vi "CRYCalc Wave & Value Unit.vi"(8 "Work in":u16(slide), 9 "Operator":u16(ring) items=["+", "--", "x", "/"], 10 "Value in":T1={"Name"="", "Curve"=[], "X data"=1, "Y data"=1, "Z data"=1, "X axis"=0, "Y axis"=1, "Z axis"=1, "X unit"="Hz", "Y unit"="", "Z unit"="deg.", "X dB ref"=1.0, "Y dB ref"=1.0, "Z dB ref"=1.0, "single val"=FALSE, "protected"=FALSE, "display X"=TRUE, "display Y"=TRUE, "display Z"=TRUE, "Test Info"="", "Step No."=0, "Plot Settings"={"Color"=0, "Interpolation"=0, "Point Style"=0, "Line Style"=0, "Point Color"=0, "Line Width"=0, "Bar Plot Style"=0, "Fill To"=0}, "AutoProtect"=FALSE} {"Z data" items=["dB", "Lin"]; "X data" items=["dB", "Lin"]; "Y data" items=["dB", "Lin"]; "Z dB ref" format="%.1f"; "Z axis" items=["Log", "Lin"]; "X dB ref" format="%.1f"; "X axis" items=["Log", "Lin"]; "Y axis" items=["Log", "Lin"]; "Y dB ref" format="%.1f"; "Curve"."z" format="%.2f"; "Curve"."y" format="%.2f"; "Curve"."x" format="%.2f"}, 11 "Wave in":T2={"Waveform"={"X0"=0.0, "dX"=0.0, "Y"=[]}, "X data"=1, "Y data"=1, "Y axis"=1, "X unit"="s", "Y unit"="V", "Y dB ref"=1.0, "display Y"=TRUE, "display X"=TRUE, "Overload?"=FALSE, "Test Info"="", "Step No."=0, "Name"="", "protected"=FALSE, "Sqc history"=[], "Signal Channel ID"=0, "Plot Settings"={"Color"=0, "Interpolation"=0, "Point Style"=0, "Line Style"=0, "Point Color"=0, "Line Width"=0, "Bar Plot Style"=0, "Fill To"=0}, "AutoProtect"=FALSE} {"Y dB ref" format="%.1f"; "Y axis" items=["Log", "Lin"]; "Y data" items=["dB", "Lin"]; "X data" items=["dB", "Lin"]}) -> (0 "Y dB ref":dbl, 1 "Y data":u16, 2 "X unit":string, 3 "Y unit":string)   [LabVIEW 2013]
uses:
  Typedef Control/CRYWaveform Cluster.ctl
  Typedef Control/CRYData Cluster.ctl
  CRYPost Processing Global.vi
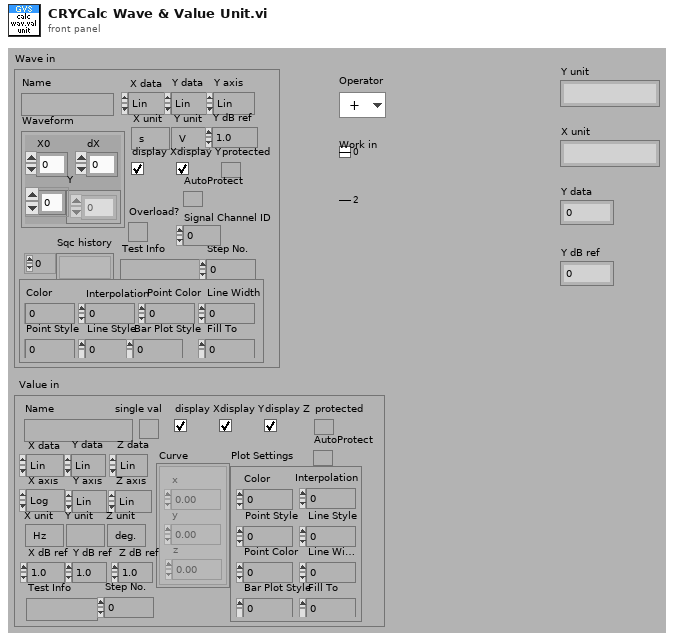
[diagram p1: front panel]
types:
  T1 = typedef "CRYData Cluster.ctl" = cluster{"Name":string, "Curve":cluster{"x":dbl, "y":dbl, "z":dbl}[], "X data":u16, "Y data":u16, "Z data":u16, "X axis":u16, "Y axis":u16, "Z axis":u16, "X unit":string, "Y unit":string, "Z unit":string, "X dB ref":dbl, "Y dB ref":dbl, "Z dB ref":dbl, "single val":bool, "protected":bool, "display X":bool, "display Y":bool, "display Z":bool, "Test Info":string, "Step No.":i32, "Plot Settings":cluster{"Color":u32, "Interpolation":u8, "Point Style":u8, "Line Style":u8, "Point Color":u32, "Line Width":u8, "Bar Plot Style":u8, "Fill To":i16}, "AutoProtect":bool}
  T2 = typedef "CRYWaveform Cluster.ctl" = cluster{"Waveform":cluster{"X0":dbl, "dX":dbl, "Y":sgl[]}, "X data":u16, "Y data":u16, "Y axis":u16, "X unit":string, "Y unit":string, "Y dB ref":dbl, "display Y":bool, "display X":bool, "Overload?":bool, "Test Info":string, "Step No.":i32, "Name":string, "protected":bool, "Sqc history":string[], "Signal Channel ID":i32, "Plot Settings":cluster{"Color":u32, "Interpolation":u8, "Point Style":u8, "Line Style":u8, "Point Color":u32, "Line Width":u8, "Bar Plot Style":u8, "Fill To":i16}, "AutoProtect":bool}
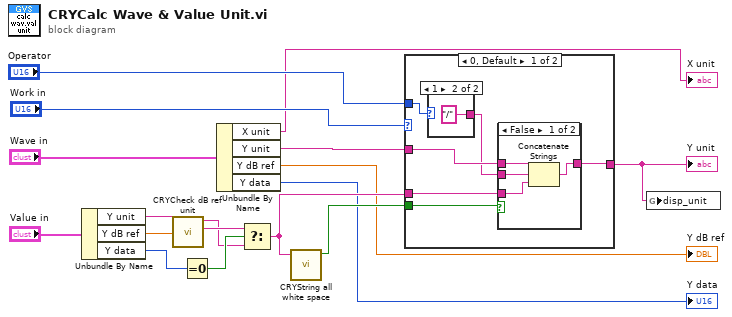
[diagram p0: block diagram]
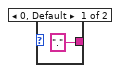
[diagram p3: hidden frame]
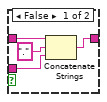
[diagram p7: hidden frame]
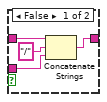
[diagram p8: hidden frame]
diagram:
  n1 = Unbundle By Name("Value in") -> ("Y unit"=w15:string, "Y dB ref"=w14:dbl, "Y data"=w12:u16)
  n2 = call "CRYCheck dB ref unit.vi"("dB ref in"=w14, "Unit in"=w15) -> ("Lin unit out"=w13:string, "Unit out"=w10:string)  [unwired: 8 out]
  n3 = Equal To 0?(x=w12) -> (x = 0?=w11:bool)
  n4 = Unbundle By Name("Wave in") -> ("X unit"=→"X unit":string, "Y unit"=w7:string, "Y dB ref"=→"Y dB ref":dbl, "Y data"=→"Y data":u16)
  n5 = Select(t=w13, s=w11, f=w10) -> (s? t:f=w6:string)
  n6 = call "CRYString all white space.vi"("String"=w6) -> ("Nothing but white space?"=w5:bool)  [unwired: 10 in]
  n7 = case shown="0, Default" "Work in" {
    tunnel: "Operator" -> [w23 w35]
    tunnel: w7 -> [w22 w34]
    tunnel: w6 -> [w19 w31]
    tunnel: [w21 w33] -> w1
    tunnel: w5 -> [w18 w32]
    frame 0, Default {
      n8 = case shown="1" w23 {
        tunnel: ["." ("string") "/" ("string")] -> w20
        frame 0, Default {
        }
        frame 1 {
        }
      }
      n9 = case shown="False" w18 {
        tunnel: w22 -> [w27 w28]
        tunnel: [w24 w28] -> w21
        tunnel: w20 -> [w26 _]
        tunnel: w19 -> [w25 _]
        frame False {
          n10 = Concatenate Strings(w27, w26, w25) -> (w24:string)
        }
        frame True {
        }
      }
    }
    frame 1, 2 {
      n11 = case shown="3" w35 {
        tunnel: w34 -> [w36 w39 w47]
        tunnel: [w36 w38 w46] -> w33
        tunnel: w32 -> [_ w40 w49]
        tunnel: w31 -> [_ w37 w48]
        frame 0, 1, Default {
        }
        frame 2 {
          n12 = case shown="True" w40 {
            tunnel: w39 -> [w44 w45]
            tunnel: [w41 w45] -> w38
            tunnel: w37 -> [w43 _]
            frame False {
              n13 = Concatenate Strings(w44, "." ("string"), w43) -> (w41:string)
            }
            frame True {
            }
          }
        }
        frame 3 {
          n14 = case shown="True" w49 {
            tunnel: w47 -> [w53 w54]
            tunnel: [w50 w54] -> w46
            tunnel: w48 -> [w52 _]
            frame False {
              n15 = Concatenate Strings(w53, "/" ("string"), w52) -> (w50:string)
            }
            frame True {
            }
          }
        }
      }
    }
  }
  "Y unit" <- w1
  n16 = global write "CRYPost Processing Global.vi" "disp_unit"(w1) -> ()
